vi "Close Server.vi"(8 "error in (no error)":errorcluster, 11 "OPC UA":T1 {"OPC tags"."data type" items=["Boolean"=1, "SByte"=2, "Byte"=3, "Int16"=4, "UInt16"=5, "Int32"=6, "UInt32"=7, "Int64"=8, "UInt64"=9, "Float"=10, "Double"=11, "String"=12, "DateTime"=13, "ByteString"=15, "Array of Boolean"=101, "Array of SByte"=102, "Array of Byte"=103, "Array of Int16"=104, "Array of UInt16"=105, "Array of Int32"=106, "Array of UInt32"=107, "Array of Int64"=108, "Array of UInt64"=109, "Array of Float"=110, "Array of Double"=111, "Array of String"=112, "Array of DateTime"=113, "Array of ByteString"=115, "Matrix of Boolean"=201, "Matrix of SByte"=202, "Matrix of Byte"=203, "Matrix of Int16"=204, "Matrix of UInt16"=205, "Matrix of Int32"=206, "Matrix of UInt32"=207, "Matrix of Int64"=208, "Matrix of UInt64"=209, "Matrix of Float"=210, "Matrix of Double"=211, "Matrix of String "=212, "Matrix of DateTime"=213, "Matrix of ByteString"=215]}) -> (0 "error out":errorcluster)   [LabVIEW 2019, in "OPC addons.lvlib"]
uses:
  OPC addons.lvlib
  OPC UA Server.ctl
  <vilib>/OPCUA/controls/OPC UA Server Refnum.ctl
  <vilib>/OPCUA/controls/NodeId.ctl
  OPC tag.ctl
  <vilib>/OPCUA/controls/Data Type.ctl
  Access level.ctl
  Period.ctl
  <vilib>/OPCUA/controls/Condition Type.ctl
  <vilib>/OPCUA/NI OPC UA Server.lvlib
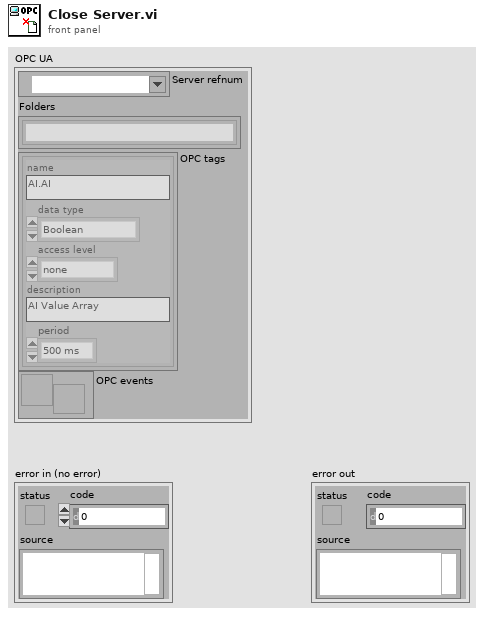
[diagram p1: front panel]
types:
  T1 = typedef "OPC addons.lvlib/OPC UA Server.ctl" = cluster{"Server refnum":T2, "Folders":T3[], "OPC tags":T4[], "OPC events":refnum<user-event>}
  T2 = typedef "OPC UA Server Refnum.ctl" = refnum<k21>
  T3 = typedef "NodeId.ctl" = string
  T4 = typedef "OPC addons.lvlib/OPC tag.ctl" = cluster{"name":string, "data type":T5, "access level":T6, "description":string, "period":T7}
  T5 = typedef "Data Type.ctl" = u16
  T6 = typedef "OPC addons.lvlib/Access level.ctl" = enum16{"none", "read-only", "write-only", "read/write"}
  T7 = typedef "OPC addons.lvlib/Period.ctl" = enum16{"on_load", "100 ms", "500 ms", "1 s"}
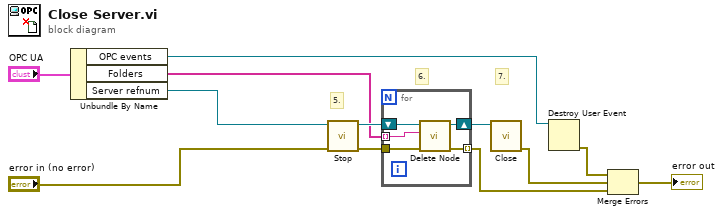
[diagram p0: block diagram]
diagram:
  # "7."
  # "6."
  # "5."
  n1 = Unbundle By Name("OPC UA") -> ("OPC events"=w6:refnum<user-event>, "Folders"=w7:T3[], "Server refnum"=w8:T2)
  n2 = call <vilib>:"Stop.vi"("error in (no error)"="error in (no error)", "OPC UA server refnum in"=w8) -> ("error out"=w10:errorcluster, "OPC UA server refnum out"=w11:T2)  [unwired: 8 in]
  n3 = for {
    tunnel: w10 -> [w16]
    tunnel: w7 -> [w15] mode=indexing
    tunnel: [w14] -> w2 mode=indexing
    shift-right: [w13] -> w12
    shift-left: w11 -> [w17]
    n4 = call <vilib>:"Delete Node.vi"("error in (no error)"=w16, "node ID"=w15, "OPC UA server refnum in"=w17) -> ("error out"=w14:errorcluster, "OPC UA server refnum out"=w13:T2)  [unwired: 7 in]
  }
  n5 = call <vilib>:"Close.vi"("OPC UA server refnum in"=w12) -> ("error out"=w3:errorcluster)  [unwired: 10 in]
  n6 = Destroy User Event(user event=w6) -> (error out=w4:errorcluster)  [unwired: 1 in]
  n7 = Merge Errors(w4, w3, w2) -> (→"error out":errorcluster)
